vi "Triggger and Read.vi"(7 "wait (ms) (20)":u32=20, 8 "error in (no error)":errorcluster, 11 "Reference in":T1={"Device"="GPIB0::4::INSTR", "Function"="", "delay"=20}) -> (0 "error out":errorcluster, 1 "value":dbl, 3 "Reference out":T1={"Device"="GPIB0::4::INSTR", "Function"="", "delay"=20}, 4 "question out":string)   [LabVIEW 2021, in "Rigol DM3052.lvlib"]
uses:
  Rigol DM3052.lvlib
  Reference.ctl
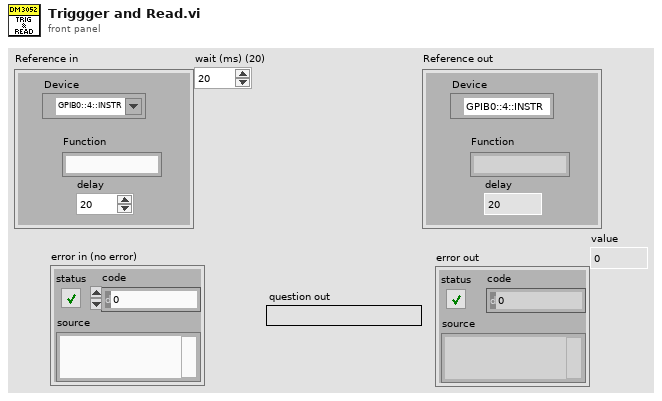
[diagram p1: front panel]
types:
  T1 = typedef "Rigol DM3052.lvlib/Reference.ctl" = cluster{"Device":refnum<visa-resource-name>, "Function":string, "delay":u32}
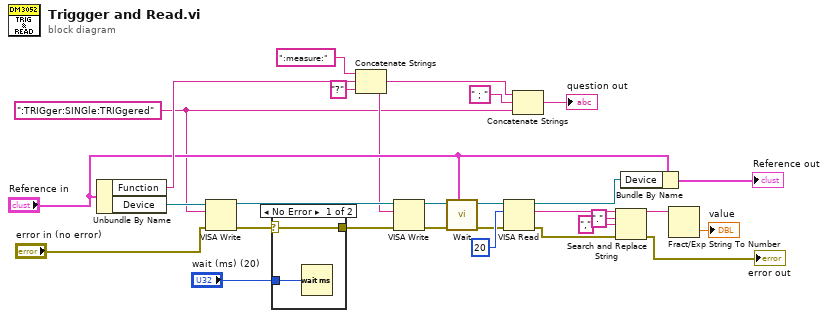
[diagram p0: block diagram]
diagram:
  w6 = ":TRIGger:SINGle:TRIGgered"
  n1 = Unbundle By Name("Reference in") -> ("Function"=w12:string, "Device"=w28:refnum<visa-resource-name>)
  n2 = VISA Write(VISA resource name=w28, write buffer=w6, error in (no error)="error in (no error)") -> (VISA resource name out=w9:refnum<visa-resource-name>, error out=w4:errorcluster)  [unwired: 1 out]
  n3 = case shown="No Error" w4 {
    selector: w4 -> [w30 w31]
    tunnel: [w30 w31] -> w3
    tunnel: "wait (ms) (20)" -> [w29 _]
    frame No Error {
      n4 = Wait (ms)(milliseconds to wait=w29) -> ()  [unwired: 1 out]
    }
    frame Error {
    }
  }
  n5 = Concatenate Strings(":measure:" ("string"), w12, "?" ("string")) -> (w7:string)
  n6 = VISA Write(VISA resource name=w9, write buffer=w7, error in (no error)=w3) -> (VISA resource name out=w15:refnum<visa-resource-name>, error out=w16:errorcluster)  [unwired: 1 out]
  n7 = call "Wait.vi"("Reference in"="Reference in", "error in (no error)"=w16, "Device in"=w15) -> ("error out"=w18:errorcluster, "Device out"=w17:refnum<visa-resource-name>)  [unwired: 7 in]
  n8 = VISA Read(VISA resource name=w17, byte count=u32 20, error in (no error)=w18) -> (VISA resource name out=w8:refnum<visa-resource-name>, read buffer=w19:string, error out=w23:errorcluster)  [unwired: 1 out]
  n9 = Concatenate Strings(w7, " ; " ("string"), w6) -> (→"question out":string)
  n10 = Search and Replace String(input string=w19, search string=".", replace string="," ("replace string (\"\")"), error in=w23) -> (result string=w22:string, error out=→"error out":errorcluster)  [unwired: 4 in, 2 out]
  n11 = Bundle By Name(cluster="Reference in", "Device"=w8) -> (→"Reference out":T1)
  n12 = Fract/Exp String To Number(string=w22) -> (number=→"value":dbl)  [unwired: 3 in, 1 out]
